vi "turret.vi"(6 "Ref Time":dbl, 8 "reinitialize? (F)":bool, 9 "Auto Target ?":bool, 11 "Yaw Control":dbl(knob)=0.10024193826887995 scale=-240.0..60.0) -> (0 "Motor Output":dbl(slide) scale=-1.0..1.0, 2 "Turret In Tol ?":bool, 3 "Turret Yaw":dbl(knob) scale=-240.0..60.0)   [LabVIEW 2011]
uses:
  <vilib>/addons/control/pid/pid.llb/PID (DBL).vi
  Robot Global Data.vi
  <vilib>/addons/control/pid/NI_PID_pid.lvlib
panel:
  in  "Motor Add CW S-Sting":dbl=-0.1
  in  "Motor Add CCW S-Sting":dbl=0.07
  in  "Motor Add CW":dbl=-0.14
  in  "Motor Add CCW":dbl=0.1
  in  "Stop Turret @+/-":dbl=0.2
  out "Table":string[][](table)
  out "Control / Stage":cluster{"Output":dbl, "Mod":i64}(graph)
  in  "Deriv 2":dbl(knob)=0.0007073415700848884 scale=0.0..0.01
  in  "Int 2":dbl(knob) scale=0.0..0.01
  in  "Prop 2":dbl(knob)=0.014855762944895264 scale=0.0..0.1
  out "Yaw Tol of Cam Err (deg)":dbl
  out "First ?":bool
  out "Robot Gyro":dbl
  out "Valid Target ?":bool
  out "PID Control":dbl
  out "Target Bearing":dbl
  in  "Max Image Turret Rate":dbl=1.0
  in  "Test Dial":dbl(knob) scale=-220.0..40.0
  in  "Max Reg Turret Rate":dbl=1.0
  in  "Yaw Tol of Cmd (deg)":dbl=1.0
  out "PID Output":dbl(graph)
  in  "Deriv":dbl(knob)=0.0003956110542098617 scale=0.0..0.01
  in  "Int":dbl(knob) scale=0.0..0.5
  in  "Prop":dbl(knob)=0.030468972393355366 scale=0.0..0.1
  out "Turret Control Response":cluster{dbl, "Turret Yaw":dbl}(graph)
  # "Fine Targeting (Camera)"
  # "P: 0.02, I: 0.00, D: 0.0006"
  # "Auto Aim FAST STL Values (TB)"
  # "P: 0.04, I: 0.003, D: 0.00128"
  # "Before Camera Image"
  # "New P=0.048"
  # "P: 0.0647, I: 0.00277, D: 0.00128"
  # "Inital Image Value"
  # "P: 0.0194, I: 0.00542, D: 0.00292"
  # "Auto Aim SLOW STL Values (TB)"
  # "Test Values"
  # "P: 0.071, I: 0.00174, D: 0.00086"
  # "P: 0.0383, I: 0.00351, D: 0.00158"
  # "Auto Aim DC Values"
  # "Need more 'P'\nfor small moves"
  # "Need some good\n'I' for small SSE, but\ncauses overshoot"
  # "More 'D' to control \nthe overshoot"
  # "Rough Targeting"
  # "DC was 0.115"
  # "STL Initial (TestBot) was 0.1"
  # "P: 0.0148, I: 0.000, D: 0.00070"
  # "Auto Aim DC Values"
  # "Low 'P' for soft\nturn landings, no \novershoot to avoid\ncamera shake"
  # "No 'I' needed since\ncamera has wide FoV\nSSE doesn't matter"
  # "Just a bit of 'D'"
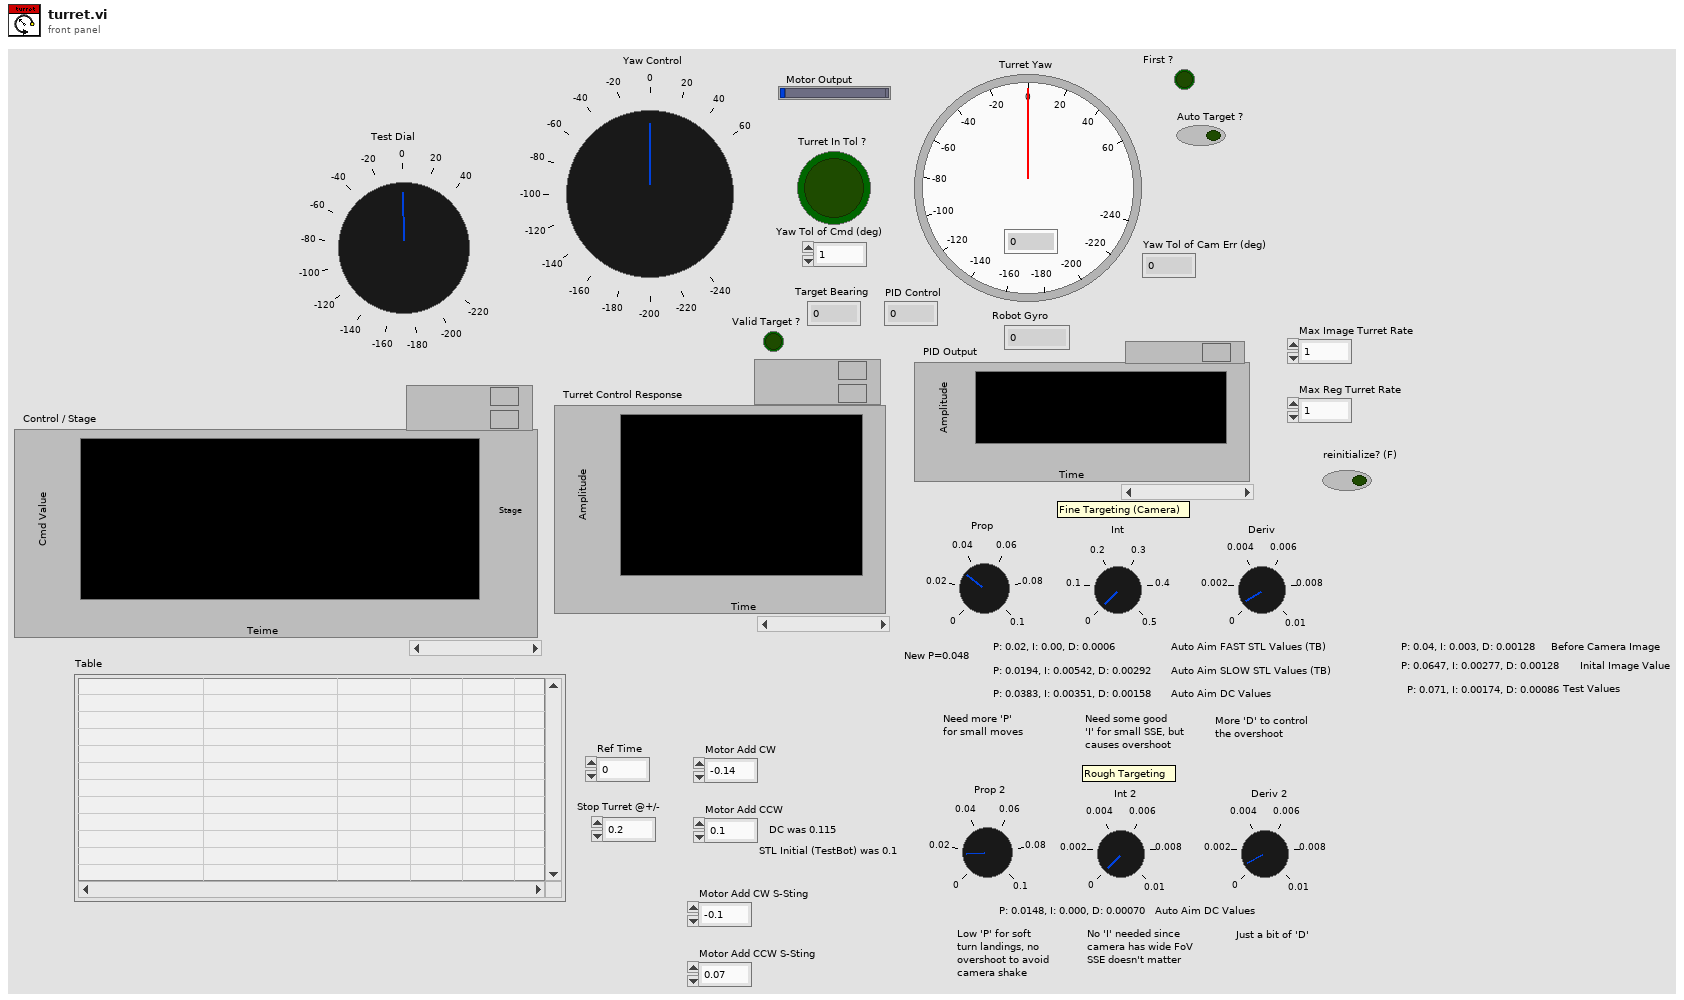
[diagram p1: front panel]
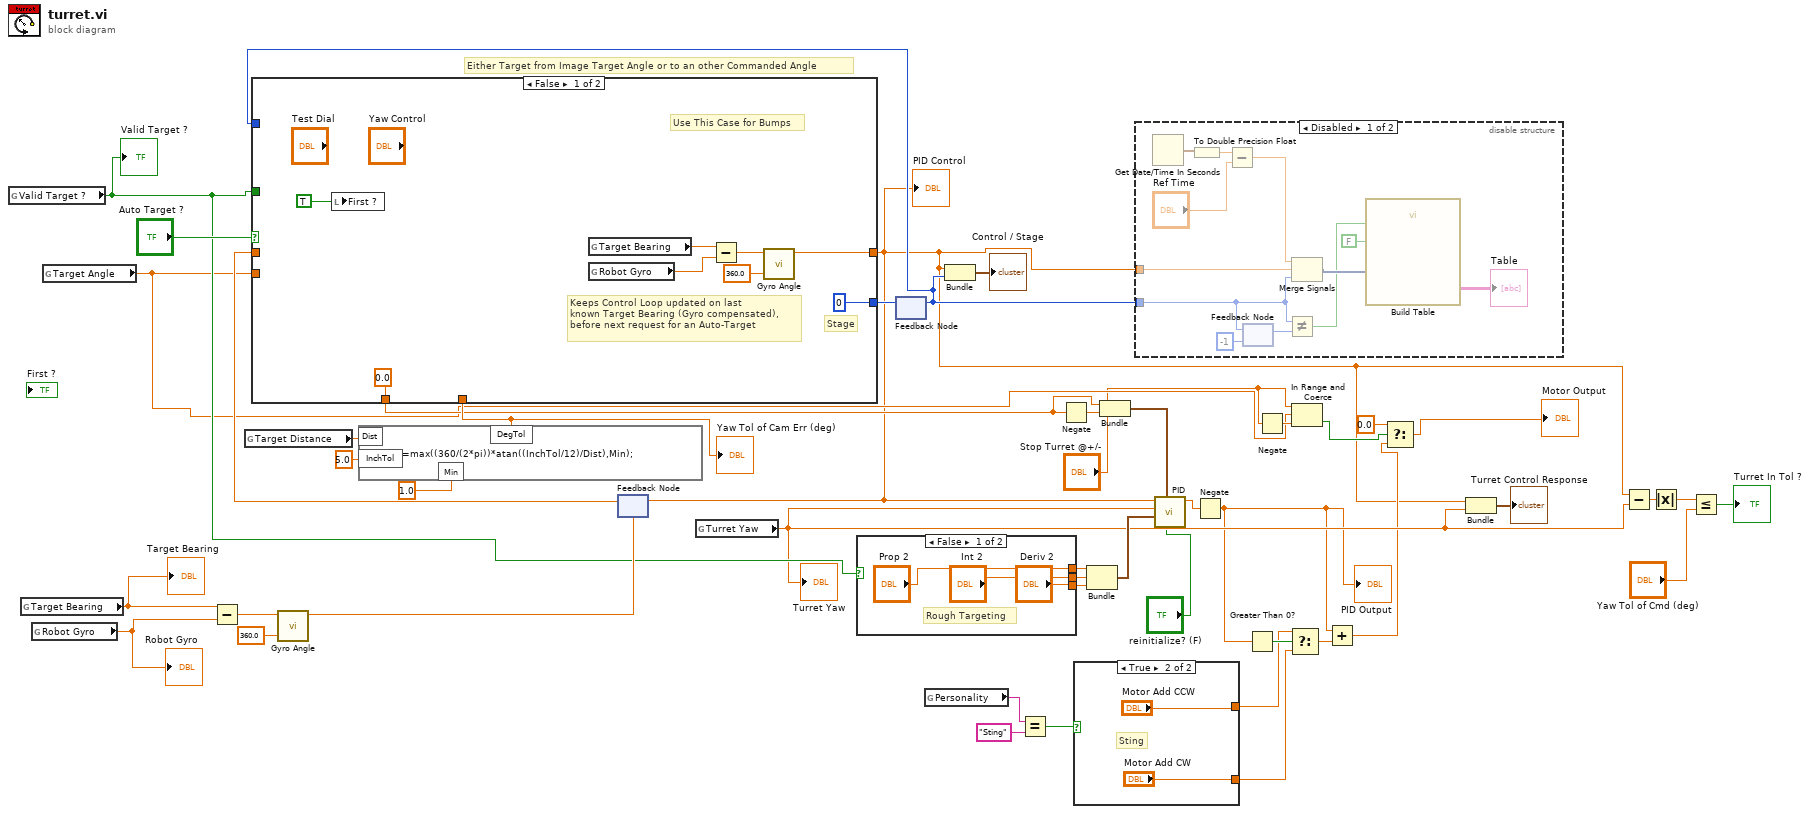
[diagram p0: block diagram]
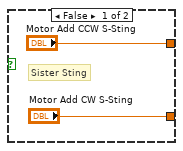
[diagram p2: hidden frame]
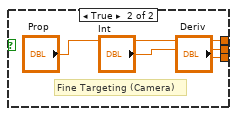
[diagram p4: hidden frame]
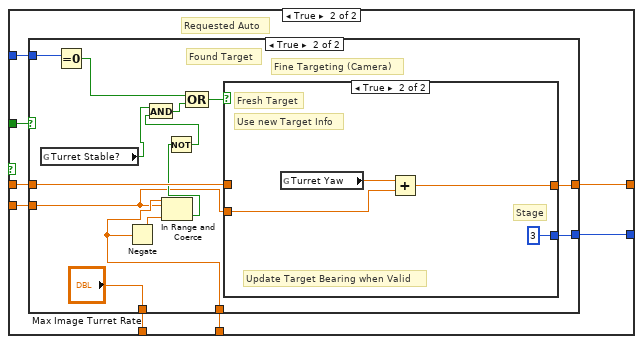
[diagram p5: hidden frame]
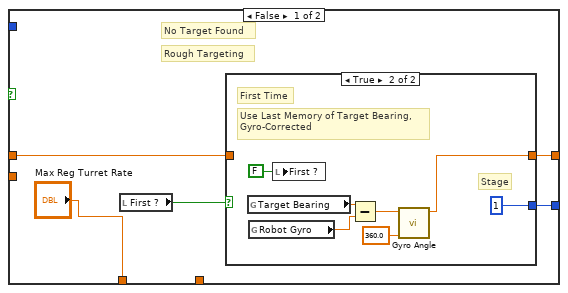
[diagram p6: hidden frame]
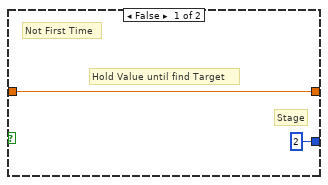
[diagram p7: hidden frame]
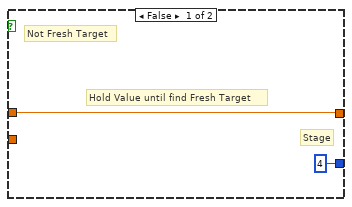
[diagram p8: hidden frame]
diagram:
  # "Either Target from Image Target Angle or to an other Commanded Angle"
  n1 = global read "Robot Global Data.vi" "Valid Target ?"() -> (w20:bool)
  "Valid Target ?" <- w20
  n2 = global read "Robot Global Data.vi" "Target Bearing"() -> (w34:dbl)
  "Target Bearing" <- w34
  n3 = global read "Robot Global Data.vi" "Robot Gyro"() -> (w14:dbl)
  "Robot Gyro" <- w14
  n4 = global read "Robot Global Data.vi" "Target Angle"() -> (w16:dbl)
  n5 = Subtract(x=w34, y=w14) -> (x-y=w33:dbl)
  n6 = global read "Robot Global Data.vi" "Target Distance"() -> (w28:dbl)
  n7 = call "Gyro Angle.vi"("Mod"=360.0, "Input"=w33) -> ("Output"=w32:dbl)  [unwired: 9 in]
  n8 = formula code="DegTol=max((360/(2*pi))*atan((InchTol/12)/Dist),Min);"("Dist"=w28, "InchTol"=5.0 ("input variable"), "Min"=1.0 ("input variable")) -> ("DegTol"=w29:dbl)
  "Yaw Tol of Cam Err (deg)" <- w29
  n9 = feedback #1(w32) -> (w35:dbl)
  n10 = global read "Robot Global Data.vi" "Turret Yaw"() -> (w12:dbl)
  "Turret Yaw" <- w12
  n11 = case shown="False" w20 {
    tunnel: ["Prop 2" "Prop"] -> w46
    tunnel: ["Deriv 2" "Deriv"] -> w45
    tunnel: ["Int 2" "Int"] -> w44
    frame False {
      # "Rough Targeting"
    }
    frame True {
      # "Fine Targeting (Camera)"
    }
  }
  n12 = feedback #2() -> (w21:i64)  [unwired: 1 in]
  n13 = case shown="False" "Auto Target ?" {
    tunnel: [w53 w67] -> w1
    tunnel: w20 -> [_ w68]
    tunnel: w35 -> [_ w66]
    tunnel: [0.0 ("Max Reg Turret Rate") w65] -> w23
    tunnel: w29 -> [_ w64]
    tunnel: [i64 0 ("Mod") w63] -> w22
    tunnel: w21 -> [_ w62]
    tunnel: w16 -> [_ w61]
    frame False {
      # "Stage"
      # "Keeps Control Loop updated on last\nknown Target Bearing (Gyro compensated),\nbefore next request for an Auto-Target"
      # "Use This Case for Bumps"
      n14 = local write "First ?"(TRUE ("First ?")) -> ()
      n15 = global read "Robot Global Data.vi" "Target Bearing"() -> (w55:dbl)
      n16 = global read "Robot Global Data.vi" "Robot Gyro"() -> (w54:dbl)
      n17 = Subtract(x=w55, y=w54) -> (x-y=w56:dbl)
      n18 = call "Gyro Angle.vi"("Mod"=360.0, "Input"=w56) -> ("Output"=w53:dbl)  [unwired: 9 in]
    }
    frame True {
      # "Requested Auto"
      n19 = case shown="True" w68 {
        tunnel: [w72 w96] -> w67
        tunnel: w66 -> [w71 w95]
        tunnel: ["Max Reg Turret Rate" "Max Image Turret Rate"] -> w65
        tunnel: w64 -> [_ w91]
        tunnel: [w69 w90] -> w63
        tunnel: w62 -> [_ w85]
        tunnel: w61 -> [_ w88]
        frame False {
          # "No Target Found"
          # "Rough Targeting"
          n20 = local read "First ?"() -> (w73:bool)
          n21 = case shown="True" w73 {
            tunnel: [w75 w78] -> w72
            tunnel: w71 -> [w75 _]
            tunnel: [i64 2 ("Mod") i64 1 ("Mod")] -> w69
            frame False {
              # "Stage"
              # "Hold Value until find Target"
              # "Not First Time"
            }
            frame True {
              # "Stage"
              # "Use Last Memory of Target Bearing,\nGyro-Corrected"
              # "First Time"
              n22 = global read "Robot Global Data.vi" "Target Bearing"() -> (w82:dbl)
              n23 = global read "Robot Global Data.vi" "Robot Gyro"() -> (w81:dbl)
              n24 = local write "First ?"(FALSE ("First ?")) -> ()
              n25 = Subtract(x=w82, y=w81) -> (x-y=w79:dbl)
              n26 = call "Gyro Angle.vi"("Mod"=360.0, "Input"=w79) -> ("Output"=w78:dbl)  [unwired: 9 in]
            }
          }
        }
        frame True {
          # "Found Target"
          # "Fine Targeting (Camera)"
          n27 = global read "Robot Global Data.vi" "Turret Stable?"() -> (w83:bool)
          n28 = Equal To 0?(x=w85) -> (x = 0?=w84:bool)
          n29 = Negate(x=w91) -> (-x=w94:dbl)
          n30 = In Range and Coerce(upper limit=w91, x=w88, lower limit=w94) -> (In Range?=w89:bool)  [unwired: 1 out]
          n31 = Not(x=w89) -> (.not. x?=w93:bool)
          n32 = And(x=w83, y=w93) -> (x .and. y?=w86:bool)
          n33 = Compound Arithmetic op=OR(w84, w86) -> (w87:bool)
          n34 = case shown="True" w87 {
            tunnel: [w98 w101] -> w96
            tunnel: w95 -> [w98 _]
            tunnel: w88 -> [_ w100]
            tunnel: [i64 4 ("Mod") i64 3 ("Mod")] -> w90
            frame False {
              # "Stage"
              # "Hold Value until find Fresh Target"
              # "Not Fresh Target"
            }
            frame True {
              # "Stage"
              # "Use new Target Info"
              # "Fresh Target"
              # "Update Target Bearing when Valid"
              n35 = global read "Robot Global Data.vi" "Turret Yaw"() -> (w102:dbl)
              n36 = Add(x=w102, y=w100) -> (x+y=w101:dbl)
            }
          }
        }
      }
    }
  }
  "PID Control" <- w1
  n37 = feedback-in #1(w1) -> ()
  n38 = feedback-in #2(w22) -> ()
  n39 = global read "Robot Global Data.vi" "Personality"() -> (w4:string)
  n40 = Bundle("Output"=w1, "Mod"=w21) -> (→"Control / Stage":cluster{"Output":dbl, "Mod":i64})  [unwired: 1 out]
  n41 = Equal?(x=w4, y="Sting") -> (x = y?=w2:bool)
  n42 = Negate(x=w23) -> (-x=w42:dbl)
  n43 = case shown="True" w2 {
    tunnel: ["Motor Add CCW S-Sting" "Motor Add CCW"] -> w9
    tunnel: ["Motor Add CW S-Sting" "Motor Add CW"] -> w8
    frame False {
      # "Sister Sting"
    }
    frame True {
      # "Sting"
    }
  }
  n44 = Bundle("Prop"=w46, "Int"=w44, "Deriv"=w45) -> (w43:cluster{"Prop":dbl, "Int":dbl, "Deriv":dbl})  [unwired: 1 out]
  n45 = Bundle("Max Image Turret Rate"=w23, w42) -> (w36:cluster{"Max Image Turret Rate":dbl, dbl})  [unwired: 1 out]
  n46 = disable-structure shown="Disabled" {
    disable-tunnel: w1 -> [w118 _]
    disable-tunnel: w21 -> [w117 _]
    frame Disabled {
      n47 = Get Date/Time In Seconds() -> (seconds since 1Jan1904=w115:timestamp)
      n48 = To Double Precision Float(number=w115) -> (double precision float=w114:dbl)
      n49 = Subtract(x=w114, y="Ref Time") -> (x-y=w113:dbl)
      n50 = feedback #3(i64 -1 ("Mod")) -> (w109:i64)
      n51 = feedback-in #3(w117) -> ()
      n52 = Not Equal?(x=w117, y=w109) -> (x != y?=w108:bool)
      n53 = Merge Signals(w113, w118, w117) -> (w116:dynamicdata)
      n54 = call "Build Table"("Include time data"=FALSE, "Enable"=w108, "Signals"=w116) -> ("Table"=→"Table":string[][])  [unwired: 2 in, 6 out]
    }
    frame Enabled {
    }
  }
  n55 = call-poly <vilib>:"PID.vi"("reinitialize? (F)"="reinitialize? (F)", "output range"=w36, "PID gains"=w43, "process variable"=w12, "setpoint"=w1) -> ("output"=w25:dbl)  [unwired: 1 in, 5 out]
  n56 = Negate(x=w25) -> (-x=w5:dbl)
  "PID Output" <- w5
  n57 = Greater Than 0?(x=w5) -> (x > 0?=w10:bool)
  n58 = Negate(x="Stop Turret @+/-") -> (-x=w17:dbl)
  n59 = Select(t=w9, s=w10, f=w8) -> (s? t:f=w7:dbl)
  n60 = In Range and Coerce(upper limit="Stop Turret @+/-", x=w16, lower limit=w17) -> (In Range?=w18:bool)  [unwired: 1 out]
  n61 = Add(x=w5, y=w7) -> (x+y=w6:dbl)
  n62 = Select(t=0.0, s=w18, f=w6) -> (s? t:f=→"Motor Output":dbl)
  n63 = Bundle("Output"=w1, "Turret Yaw"=w12) -> (→"Turret Control Response":cluster{"Output":dbl, "Turret Yaw":dbl})  [unwired: 1 out]
  n64 = Subtract(x=w1, y=w12) -> (x-y=w40:dbl)
  n65 = Absolute Value(x=w40) -> (abs(x)=w37:dbl)
  n66 = Less Or Equal?(x=w37, y="Yaw Tol of Cmd (deg)") -> (x <= y?=→"Turret In Tol ?":bool)
